vi "Transfer function VI example.vi"() -> ()   [LabVIEW 2019]
uses:
  <vilib>/addons/Control Design/_Model Construction/Model Creation.llb/Model Creation SubVI/cd_Create Transfer Function Model.vi
  <vilib>/addons/Control Design/_Model Conversions/Model Type.llb/Model Conversion SubVI/cd_Convert Transfer Function to Zero-Pole-Gain Model.vi
  <vilib>/addons/Control Design/_Utility/Model Viewer.llb/Model Viewer SubVI/cd_Draw Zero-Pole-Gain Equation (ZPK).vi
  <vilib>/addons/Control Design/_Dynamic Analysis/Dynamic Analysis.llb/Dynamic Analysis subVI/cd_Pole-Zero Map (Transfer Function).vi
  <vilib>/addons/Control Design/_Utility/Model Viewer.llb/Model Viewer SubVI/cd_Draw Transfer Function Equation (TF).vi
  <vilib>/addons/Control Design/_Model Construction/NI_LinSys_Model Creation.lvlib
  <vilib>/addons/Control Design/_Utility/NI_CD_Model Viewer.lvlib
  <vilib>/addons/Control Design/_Dynamic Analysis/NI_CD_Dynamic Analysis.lvlib
  <vilib>/addons/Control Design/_Model Conversions/NI_CD_Model Type.lvlib
panel:
  out "Zero-Pole-Gain Model":picture
  out "Zeros":cdb[](array[numeric]) format="%.4f"
  out "Poles":cdb[](array[numeric]) format="%.4f"
  out "Pole-Zero Map":cluster{dbl[], dbl[]}[](graph)
  out "Transfer function":picture
  in  "Numerator":dbl[](array[numeric]) format="%#.5g"
  in  "Denominator":dbl[](array[numeric]) format="%#.5g"
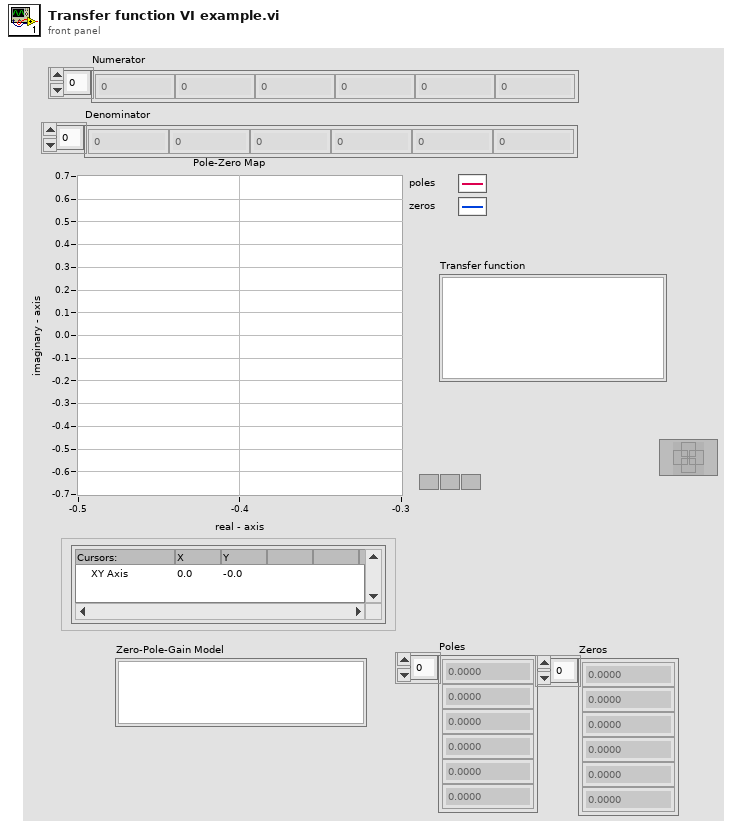
[diagram p1: front panel]
types:
  T1 = typedef "NI_LinSys_Model Typedefs.lvlib/CD Transfer Function Model (MIMO).ctl" = cluster{"properties":T2, "transfer function(s)":T3[][]}
  T2 = typedef "NI_LinSys_Model Typedefs.lvlib/CD General Elements.ctl" = cluster{"Model name":string, "Input names":string[], "Output names":string[], "Input Delays":dbl[], "Output Delays":dbl[], "Sampling Time":dbl, "Notes":string}
  T3 = typedef "NI_LinSys_Model Typedefs.lvlib/CD Transfer Function Model (SISO).ctl" = cluster{"Numerator":dbl[], "Denominator":dbl[], "delay":dbl}
  T4 = typedef "NI_LinSys_Model Typedefs.lvlib/CD Zero-Pole-Gain Model (MIMO).ctl" = cluster{"properties":T2, "zero-pole-gain(s)":T5[][]}
  T5 = typedef "NI_LinSys_Model Typedefs.lvlib/CD Zero-Pole-Gain Model (SISO).ctl" = cluster{"Gain":dbl, "Zeros":cdb[], "Poles":cdb[], "delay":dbl}
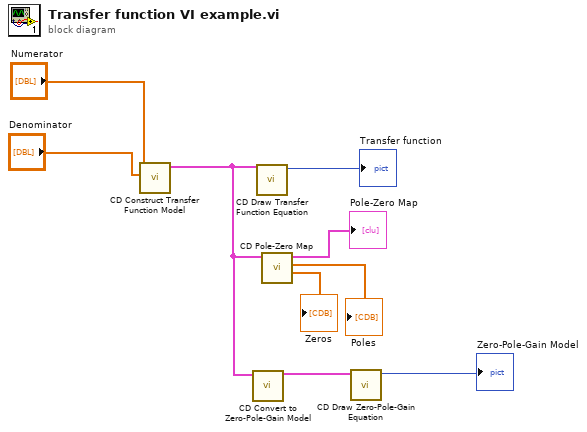
[diagram p0: block diagram]
diagram:
  n1 = call-poly <vilib>:"CD Construct Transfer Function Model.vi"("Denominator"="Denominator", "Numerator"="Numerator") -> ("Transfer Function Model"=w2:T1)  [unwired: 8 in, 1 out]
  n2 = call-poly <vilib>:"CD Convert to Zero-Pole-Gain Model.vi"("Transfer Function Model"=w2) -> ("Zero-Pole-Gain Model"=w1:T4)  [unwired: 9 in, 1 out]
  n3 = call-poly <vilib>:"CD Draw Transfer Function Equation.vi"("Transfer Function Model"=w2) -> ("Equation"=→"Transfer function":picture)  [unwired: 8 in, 2 out]
  n4 = call-poly <vilib>:"CD Pole-Zero Map.vi"("Transfer Function Model"=w2) -> ("Zeros"=→"Zeros":cdb[], "Poles"=→"Poles":cdb[], "Pole-Zero Map"=→"Pole-Zero Map":cluster{dbl[], dbl[]}[])  [unwired: 7 in, 1 out]
  n5 = call-poly <vilib>:"CD Draw Zero-Pole-Gain Equation.vi"("Zero-Pole-Gain Model"=w1) -> ("Equation"=→"Zero-Pole-Gain Model":picture)  [unwired: 8 in, 2 out]
